vi "7915_p2p_IQ_gen_1_92GHz_8+4.vi"() -> ()   [LabVIEW 2021]
uses:
  <vilib>/Platform/TimedLoop/XDataNode/timing_clust.ctl
  <vilib>/Platform/TimedLoop/XDataNode/nitl_modes.ctl
  <vilib>/Platform/TimedLoop/XDataNode/wakeup.ctl
  <vilib>/rvi/Emulation/niFpgaSctlEmulationGetInTimedLoop.vi
  <vilib>/rvi/Emulation/niFpgaEmulationReportErrorSimple.vi
  <vilib>/rvi/Emulation/niFpgaGetClockAttributes.vi
  <vilib>/rvi/Emulation/niFpgaCriticalErrorInLSC.vi
  <vilib>/rvi/interface/RandomDataEmulation/nirviRandomDataMultiElementFPGAFIFO.vi
  <instcachedir>/0/nirviRandomDataMultiElementFPGAFIFO_3E9965BA1FAD4E7B8DABA31768A09B1F.lvgen/nirviRandomDataMultiElementFPGAFIFO_3E9965BA1FAD4E7B8DABA31768A09B1F_000.vi
  <vilib>/rvi/interface/RandomDataEmulation/niFpgaRandomDataHandleErrors.vi
  <instrlib>/_niInstr/Basic Elements/v1/FPGA/Private/Count Up U32.vi
  <vilib>/Platform/TimedLoop/XDataNode/XDataNode.xnode
  <vilib>/rvi/DataTransferAndStorage/Container/XNode/niFpgaContainer.xnode
  <vilib>/rvi/FIFO/Fifo_Resource/nirvififoEmulationP2P.vi
  <vilib>/rvi/interface/RandomDataEmulation/nirviRandomDataFpgaMultiElementTemplate.vi
  <vilib>/Platform/TimedLoop/XDataNode/XDNodeRunTimeDep.lvlib
  <instrlib>/_niInstr/Basic Elements/v1/FPGA/niInstr Basic Elements v1 FPGA.lvlib
panel:
  out "lost sampels":u32
  in  "P2P empty room for runing":u32=2000
  out "pulse TX status":T1
  in  "reset system clock":bool
  # "Data Path Configuration"
  # "AI Trigger Configuration"
  # "AI Stream Configuration"
  # "AO Stream Configuration"
  # "Module Status"
  # "AO Buffer Configuration"
  # "Device Utilization\n---------------------------\nTotal Slices: 62.6% (18977 out of 30300)\nSlice Registers: 23.8% (115206 out of 484800)\nSlice LUTs: 38.2% (92532 out of 242400)\nBlock RAMs: 56.8% (341 out of 600)\nDSP48s: 0.3% (6 out of 1920)\n\nNote: Utilization numbers are for the KU040. Exact values will vary for the KU060 and KU035."
  # "User-defined Controls"
  # "AO Trigger Configuration"
  # "Utilization numbers are for the KU060."
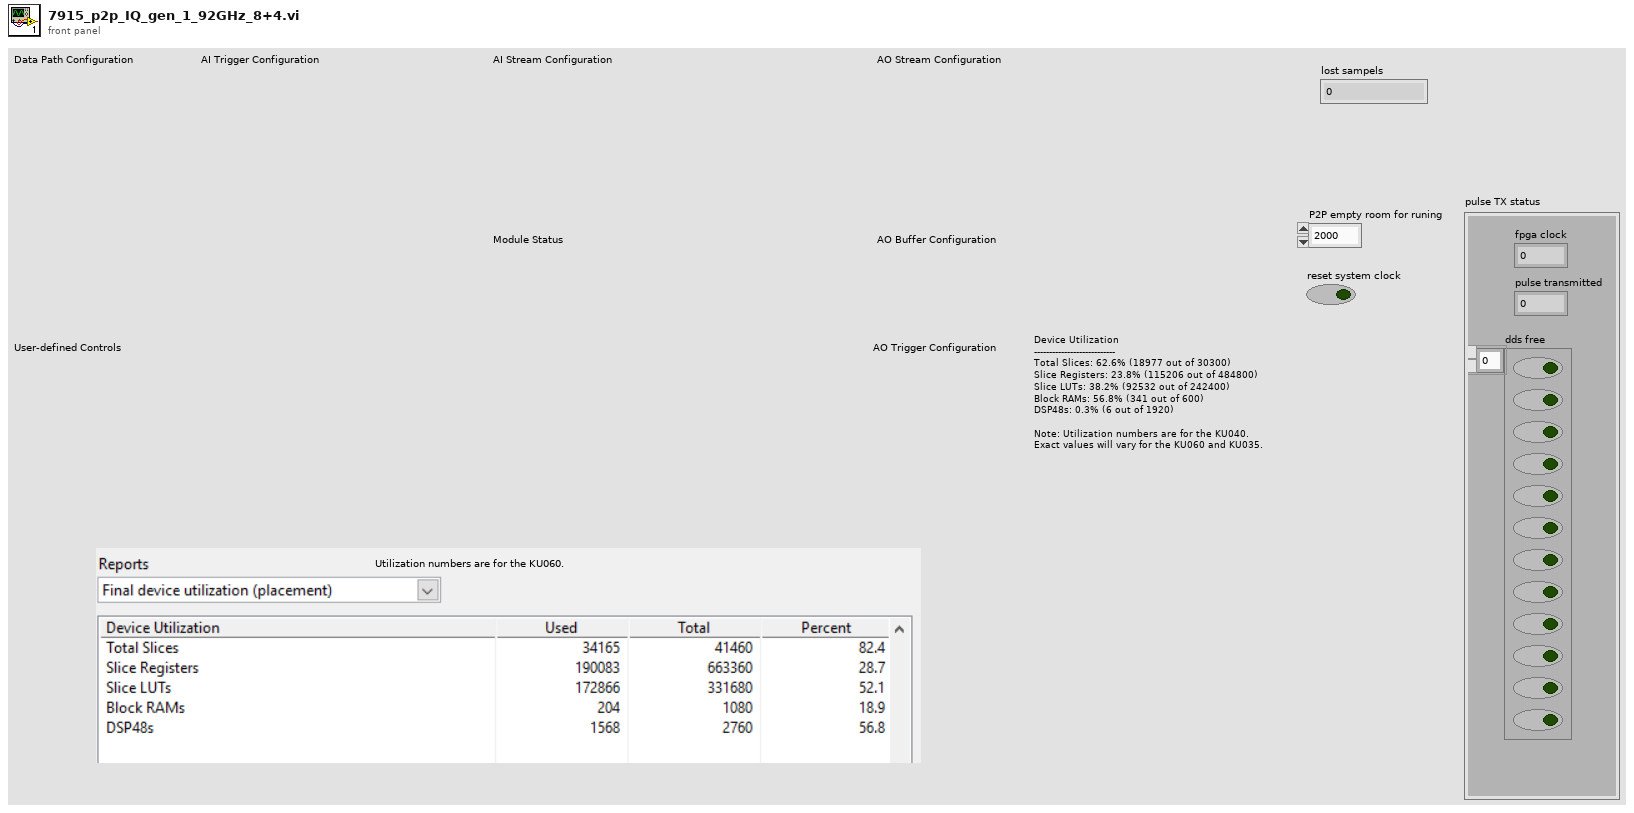
[diagram p1: front panel]
types:
  T1 = cluster{"fpga clock":u64, "pulse transmitted":u32, "dds free":bool[]}
  T2 = typedef "XDNodeRunTimeDep.lvlib/timing_clust.ctl" = cluster{"Expected End [f-1]":u64, "Actual End [f-1]":u64, "Finished Late? [f-1]":bool, "Expected End [i-1]":u64, "Actual End [i-1]":u64, "Finished Late? [i-1]":bool, "Expected Start [i]":u64, "Actual Start [i]":u64, "Expected Start [f]":u64, "Actual Start [f]":u64, "Source Name":string, "Structure Name":string, "Period":i64, "Deadline":i64, "Offset":i64, "Start":i64, "Priority":i32, "Timeout":i32, "Mode":T3, "Wakeup Reason":T4, "Error":errorcluster, "Source Type":string, "Secondary Source Type":string, "Global End Time":u64, "Global Start Time":u64, "Frame Duration":u64, "Iteration Duration":u64, "Assigned CPU":i32, "I/O Scan Engine Mode":u32}
  T3 = typedef "XDNodeRunTimeDep.lvlib/nitl_modes.ctl" = enum32{"No Change", "Process missed periods, maintain original phase", "Discard missed periods, maintain original phase", "Process missed periods, ignore original phase", "Discard missed periods, ignore original phase"}
  T4 = typedef "XDNodeRunTimeDep.lvlib/wakeup.ctl" = enum32{"Normal", "Aborted", "Asynchronous wakeup", "Timing source error", "Timed loop error", "Timeout"}
  T5 = cluster{"Memory In":refnum<k21>, "Memory In 2":refnum<k21>, "Memory In 3":refnum<k21>, "Memory In 6":refnum<k21>}
  T6 = cluster{"clock x2":refnum<k21>, "Memory In":refnum<k21>, "Memory In 2":refnum<k21>, "Memory In 3":refnum<k21>, "Memory In 4":refnum<k21>}
  T7 = typedef "niInstr DSP v1 Shared.lvlib/IQ Data.ctl" = cluster{"I":fxp<+/-,18,1>, "Q":fxp<+/-,18,1>, "overflow":bool}
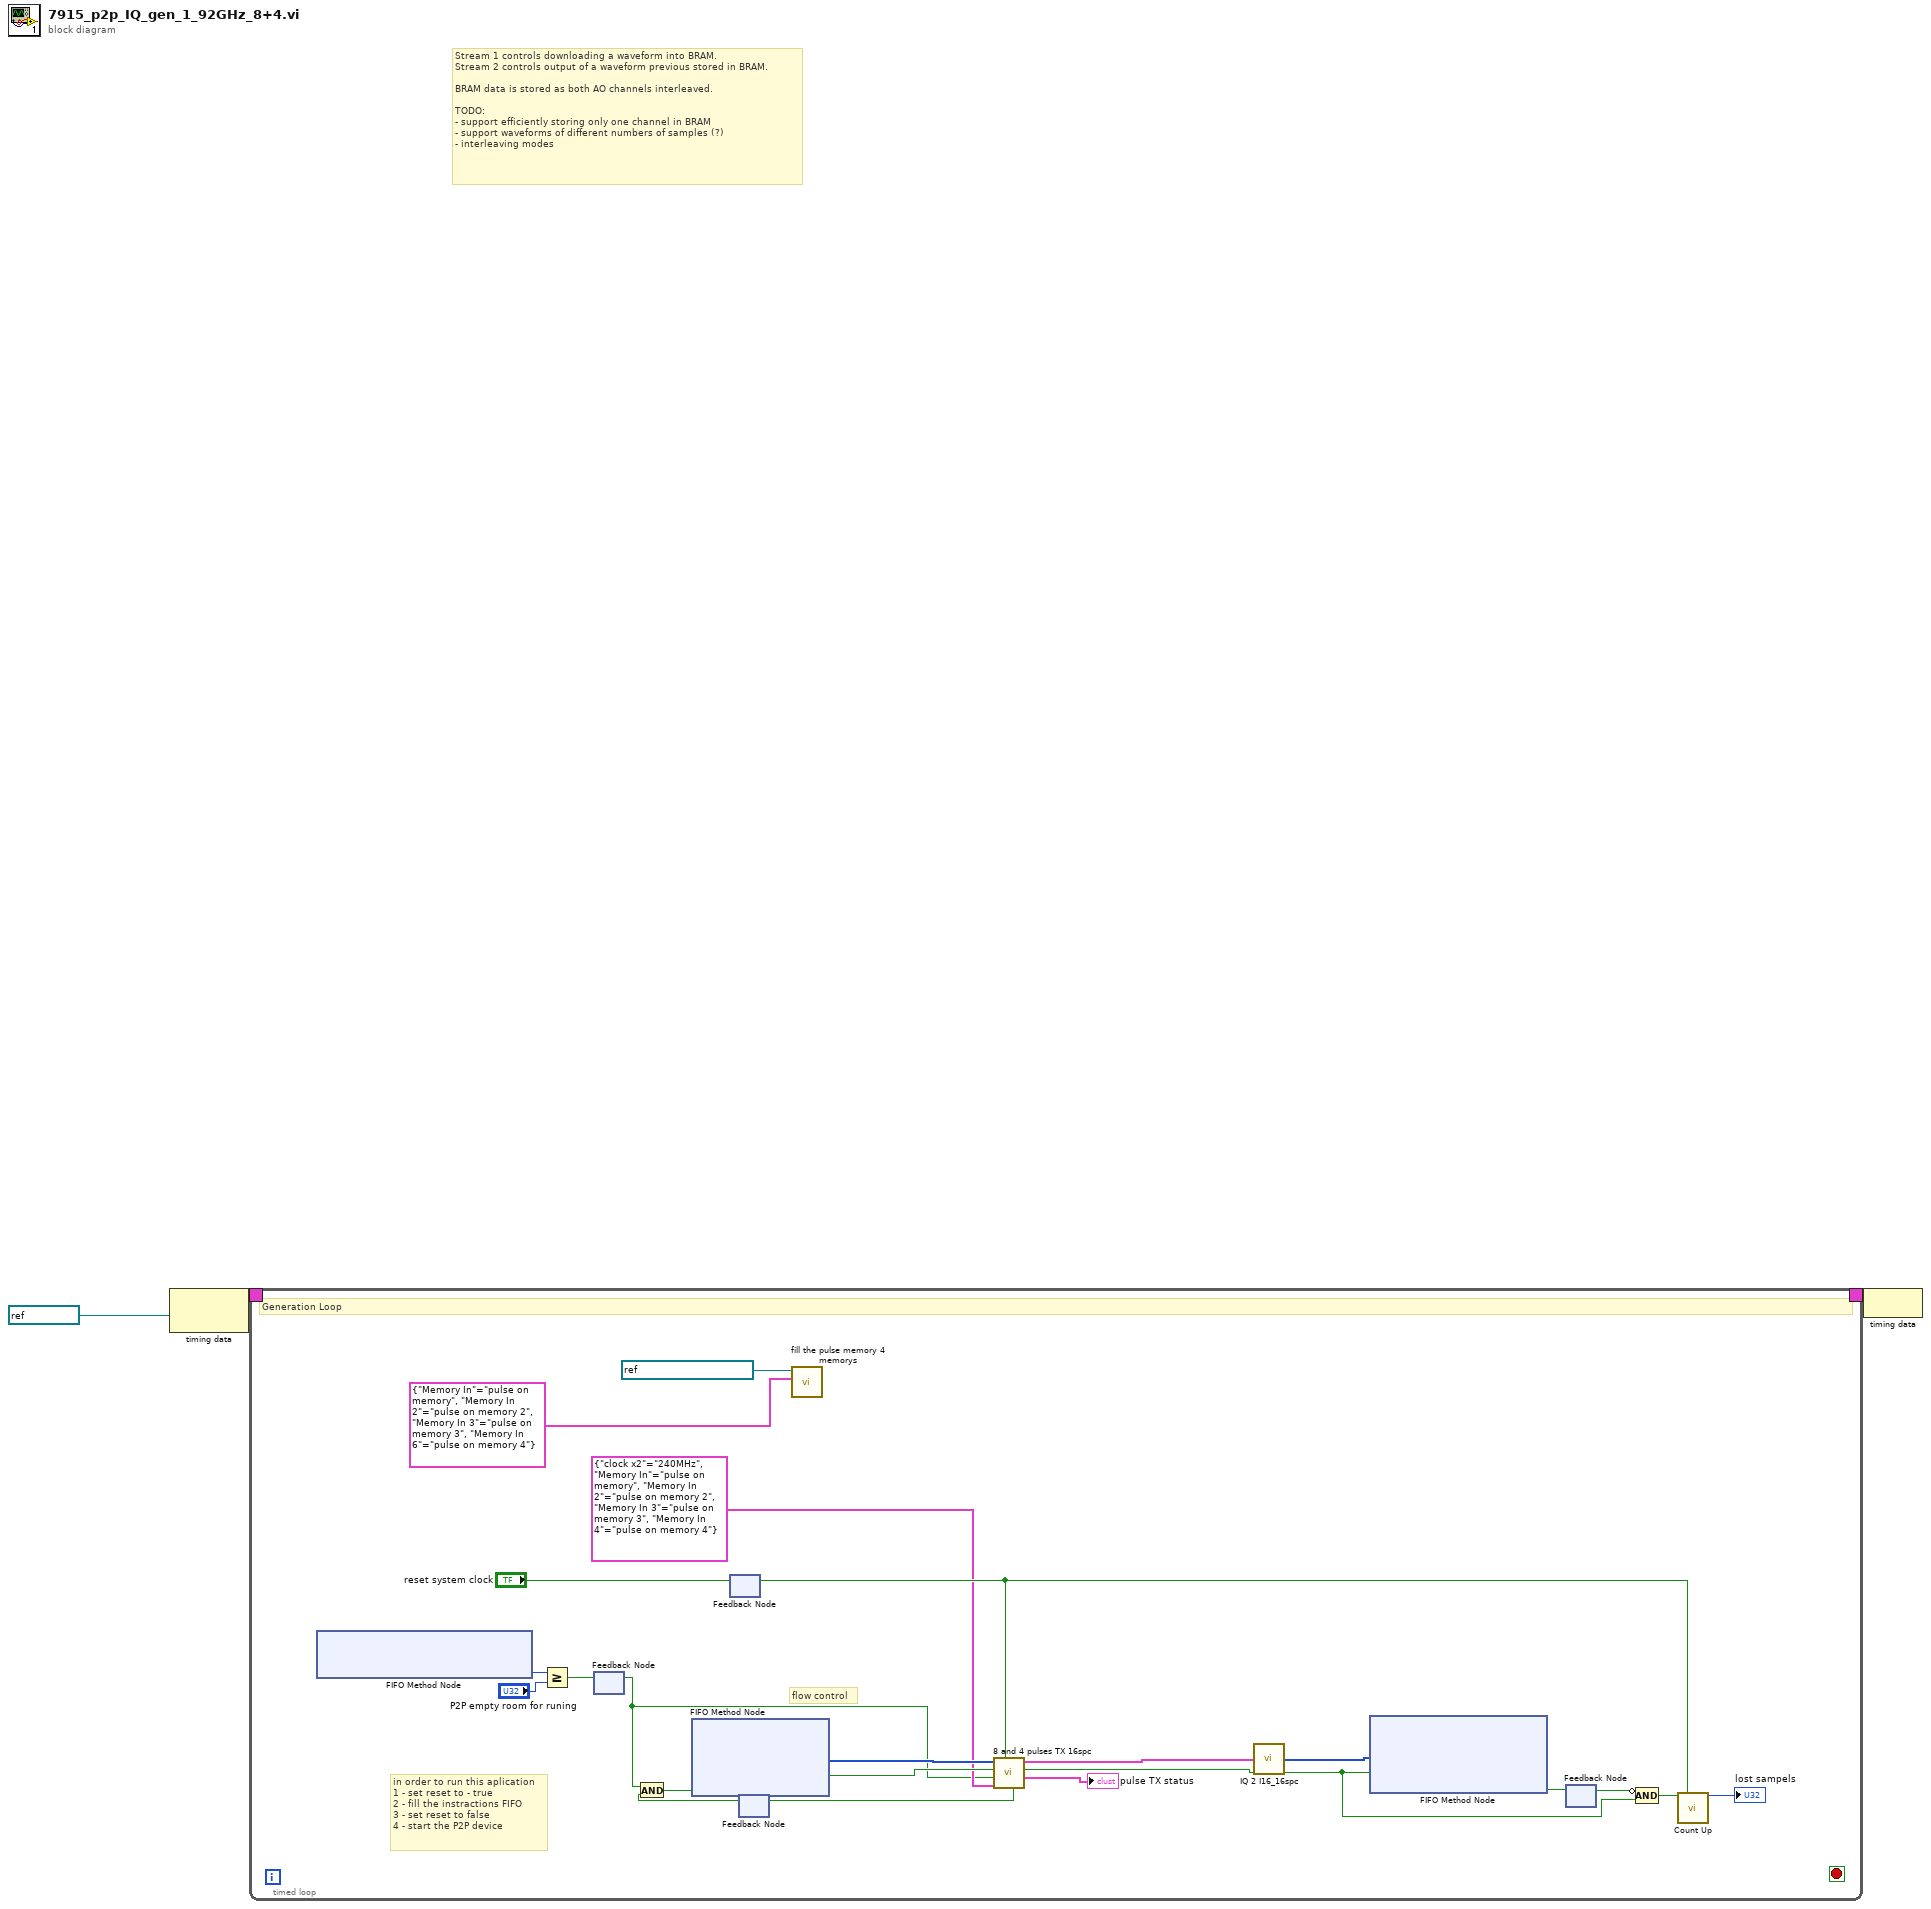
[diagram p0: block diagram]
diagram:
  # "Stream 1 controls downloading a waveform into BRAM.\nStream 2 controls output of a waveform previous stored in BRAM.\n\nBRAM data is stored as both AO channels interleaved.\n\nTODO:\n- support efficiently storing only one channel in BRAM\n- support waveforms of different numbers of samples (?)\n- interleaving modes"
  n1 = node-c288(refnum<k21> "120MHz" ("Source Name")) -> (w3:T2)
  n2 = timed-loop {
    timing: w3 -> [_]
    timing-out: [_] -> w2
    stop <- _ stop-if-true
    # "flow control"
    # "in order to run this aplication\n1 - set reset to - true\n2 - fill the instractions FIFO\n3 - set reset to false\n4 - start the P2P device"
    # "Generation Loop"
    n3 = xnode ("FIFO Method Node")() -> ("Number of Elements to Write"=w14:u32)  [unwired: 1 in, 1 out]
    n4 = Greater Or Equal?(x=w14, y="P2P empty room for runing") -> (x >= y?=w23:bool)
    n5 = feedback #1() -> (w4:bool)  [unwired: 1 in]
    n6 = feedback-in #1(w23) -> ()
    n7 = feedback-in #2("reset system clock") -> ()
    n8 = feedback #2() -> (w18:bool)  [unwired: 1 in]
    n9 = feedback #3() -> (w7:bool)  [unwired: 1 in]
    n10 = And(x=w4, y=w7) -> (x .and. y?=w6:bool)
    n11 = xnode ("FIFO Method Node")("Ready for Output"=w6) -> ("Element"=w25:u64[], "Output Valid"=w24:bool)  [unwired: 1 in, 1 out]
    n12 = call "fill the pulse memory 4 memorys.vi"("memory units"=T5 {"Memory In"="pulse on memory", "Memory In 2"="pulse on memory 2", "Memory In 3"="pulse on memory 3", "Memory In 6"="pulse on memory 4"}, "FIFO In"=refnum<k21> "fifo pulse from host") -> ()  [unwired: 10 in]
    n13 = call "8 and 4 pulses TX 16spc.vi"("reset system clock"=w18, "referenses 2"=T6 {"clock x2"="240MHz", "Memory In"="pulse on memory", "Memory In 2"="pulse on memory 2", "Memory In 3"="pulse on memory 3", "Memory In 4"="pulse on memory 4"} ("referenses"), "IQ_run"=w4, "PDW input Valid"=w24, "array PDW"=w25) -> ("pulse TX status"=→"pulse TX status":T1, "output valid"=w12:bool, "IQ out"=w13:T7[], "ready for input"=w8:bool)  [unwired: 3 in]
    n14 = feedback-in #3(w8) -> ()
    n15 = call "IQ 2 I16_16spc.vi"("IQ in"=w13) -> ("interleaved IQ array"=w16:i16[])
    n16 = xnode ("FIFO Method Node")("Element"=w16, "Input Valid"=w12) -> ("Ready for Input"=w15:bool)  [unwired: 1 in, 1 out]
    n17 = feedback-in #4(w15) -> ()
    n18 = feedback #4() -> (w21:bool)  [unwired: 1 in]
    n19 = Compound Arithmetic op=AND(invert w21, w12) -> (w20:bool)
    n20 = call-poly <instrlib>:"Count Up.vi"("increment"=w20, "reset"=w18) -> ("count out"=→"lost sampels":u32)  [unwired: 13 in]
  }
  n21 = node-c288(w2) -> ()
